vi "画模板匹配找到的矩形框.vi"(8 "Color":u32(colorbox)=16711680, 10 "Matches (Pattern Matching 1)":T2(array[cluster]), 11 "Image":T1) -> ()   [LabVIEW 2014]
uses:
  <vilib>/vision/Image Controls.llb/IMAQ Image.ctl
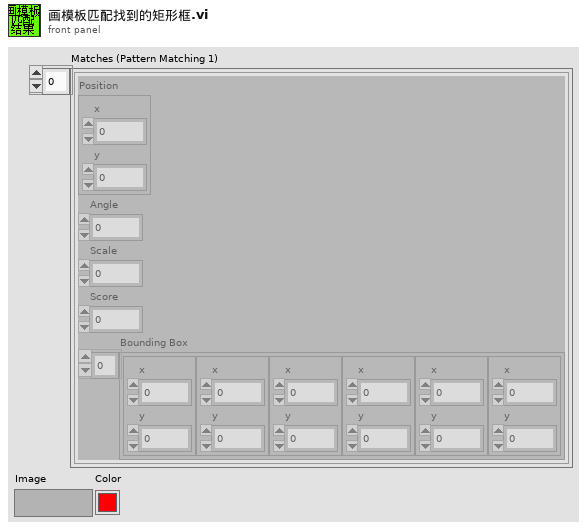
[diagram p1: front panel]
types:
  T1 = typedef "IMAQ Image.ctl" = refnum<image>
  T2 = cluster{"Position":cluster{"x":sgl, "y":sgl}, "Angle":sgl, "Scale":sgl, "Score":sgl, "Bounding Box":cluster{"x":sgl, "y":sgl}[]}[]
  T3 = cluster{"Position":cluster{"x":sgl, "y":sgl}, "Angle":sgl, "Scale":sgl, "Score":sgl, "Bounding Box":cluster{"x":sgl, "y":sgl}[]}
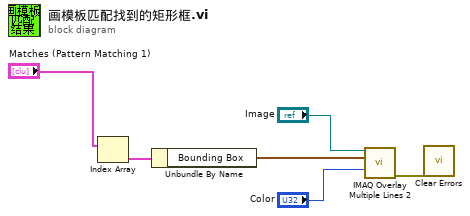
[diagram p0: block diagram]
diagram:
  n1 = Index Array(array="Matches (Pattern Matching 1)") -> (element=w6:T3)  [unwired: 1 in]
  n2 = Unbundle By Name(w6) -> ("Bounding Box"=w4:cluster{"x":sgl, "y":sgl}[])
  n3 = call "IMAQ Overlay Multiple Lines 2"("Image"="Image", "Line End Points"=w4, "Color"="Color") -> ("error out"=w1:errorcluster)  [unwired: 11 in, 1 out]
  n4 = call <vilib>:"Clear Errors.vi"("error in (no error)"=w1) -> ()  [unwired: 5 in, 2 out]
